vi "Basic Function Generator.vi"(3 "offset":dbl format="%0.2p", 4 "square wave duty cycle (%)":dbl=50.0 format="%0.2f", 5 "reset signal":bool, 6 "sampling info":cluster{"Fs":dbl, "#s":dbl}={"Fs"=1000.0, "#s"=1000.0} {"Fs" format="%.2p"}, 7 "signal type":T1(ring), 8 "error in (no error)":errorcluster, 9 "phase":dbl format="%.2p", 10 "amplitude":dbl=1.0 format="%0.2p", 11 "frequency":dbl=10.0 format="%0.2p") -> (0 "error out":errorcluster, 1 "phase out":dbl format="%.2p", 2 "signal out":waveform(dbl))   [LabVIEW 2020, in "NI_MABase.lvlib"]
doc: "Creates an output waveform based on <B>signal type</B>."
uses:
  NI_MABase.lvlib
  NI_AALBase.lvlib
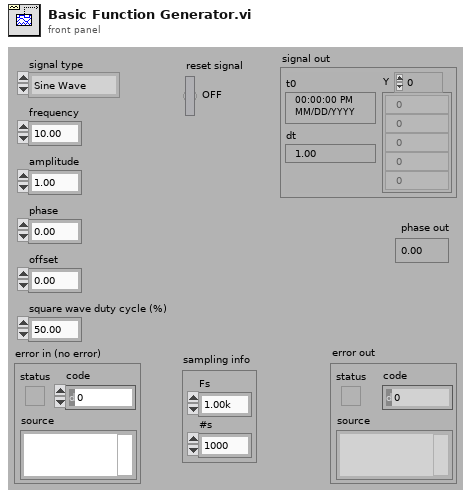
[diagram p1: front panel]
types:
  T1 = enum16{"Sine Wave", "Triangle Wave", "Square Wave", "Sawtooth Wave"}
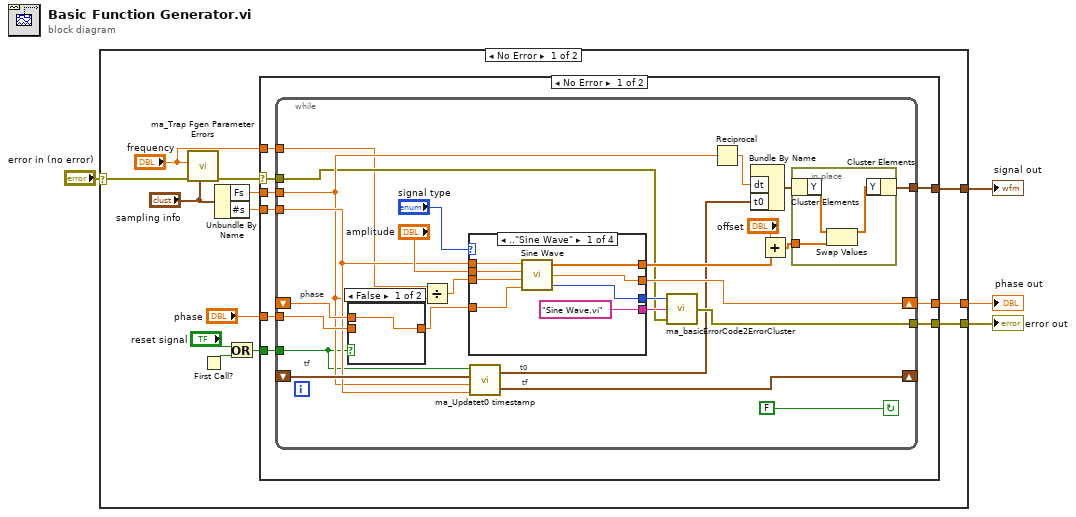
[diagram p0: block diagram]
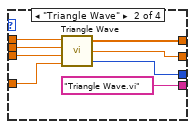
[diagram p2: hidden frame]
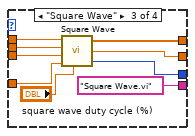
[diagram p3: hidden frame]
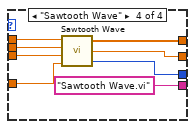
[diagram p4: hidden frame]
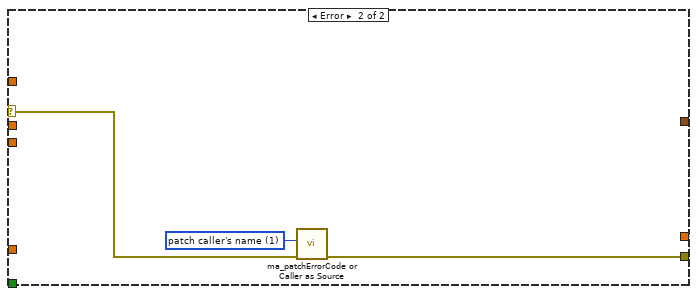
[diagram p6: hidden frame]
diagram:
  n1 = case shown="No Error" "error in (no error)" {
    selector: "error in (no error)" -> [w8 w94]
    tunnel: [w17 w94] -> w4
    tunnel: [w6 _] -> w2
    tunnel: [w5 _] -> w1
    frame No Error {
      n2 = call "ma_Trap Fgen Parameter Errors.vi"("Sampling info"="sampling info", "error in (no error)"=w8, "frequency"="frequency") -> ("error out"=w16:errorcluster)  [unwired: 8 in]
      n3 = First Call?() -> (First Call?: T/F=w11:bool)
      n4 = Unbundle By Name("sampling info") -> ("Fs"=w13:dbl, "#s"=w12:dbl)
      n5 = Or(x="reset signal", y=w11) -> (x .or. y?=w9:bool)
      n6 = case shown="No Error" w16 {
        selector: w16 -> [w20 w92]
        tunnel: [w26 w93] -> w5
        tunnel: [w25 w91] -> w17
        tunnel: "phase" -> [w24 _]
        tunnel: w13 -> [w23 _]
        tunnel: w12 -> [w22 _]
        tunnel: w9 -> [w21 _]
        tunnel: [w18 _] -> w6
        tunnel: "frequency" -> [w19 _]
        frame No Error {
          n7 = while {
            tunnel: w20 -> [w35]
            tunnel: w21 -> [w38]
            tunnel: w22 -> [w40]
            tunnel: w23 -> [w39]
            tunnel: w24 -> [w49]
            tunnel: [w34] -> w25
            shift-left: _ -> [w51]
            shift-right: [w41] -> w26
            shift-left: _ -> [w50]
            shift-right: [w29] -> _
            tunnel: w19 -> [w32]
            tunnel: [w27] -> w18
            stop <- FALSE continue-if-true
            # "tf"
            # "t0"
            # "phase"
            # "tf"
            n8 = case shown="False" w38 {
              tunnel: w51 -> [w88 _]
              tunnel: [w88 w89] -> w43
              tunnel: w49 -> [_ w89]
              frame False {
              }
              frame True {
              }
            }
            n9 = Divide(x=w32, y=w39) -> (x/y=w46:dbl)
            n10 = case shown="..\"Sine Wave\"" "signal type" {
              tunnel: w46 -> [w62 w70 w79 w87]
              tunnel: "amplitude" -> [w61 w69 w78 w86]
              tunnel: w40 -> [w60 w68 w77 w85]
              tunnel: w43 -> [w59 w67 w76 w84]
              tunnel: [w58 w66 w75 w83] -> w41
              tunnel: [w57 w65 w74 w82] -> w45
              tunnel: ["Sine Wave.vi" ("subVI Name") "Triangle Wave.vi" ("subVI Name") "Square Wave.vi" ("subVI Name") "Sawtooth Wave.vi" ("subVI Name")] -> w37
              tunnel: [w56 w64 w72 w80] -> w36
              frame .."Sine Wave" {
                n11 = call "Sine Wave.vi"("samples"=w60, "amplitude"=w61, "frequency"=w62, "phase in"=w59) -> ("sine wave"=w57:dbl[], "phase out"=w58:dbl, "error"=w56:i32)  [unwired: 1 in]
              }
              frame "Triangle Wave" {
                n12 = call "Triangle Wave.vi"("samples"=w68, "amplitude"=w69, "frequency"=w70, "phase in"=w67) -> ("triangle wave"=w65:dbl[], "phase out"=w66:dbl, "error"=w64:i32)  [unwired: 1 in]
              }
              frame "Square Wave" {
                n13 = call "Square Wave.vi"("samples"=w77, "amplitude"=w78, "frequency"=w79, "duty cycle (%)"="square wave duty cycle (%)", "phase in"=w76) -> ("square wave"=w74:dbl[], "phase out"=w75:dbl, "error"=w72:i32)  [unwired: 1 in]
              }
              frame "Sawtooth Wave" {
                n14 = call "Sawtooth Wave.vi"("samples"=w85, "amplitude"=w86, "frequency"=w87, "phase in"=w84) -> ("sawtooth wave"=w82:dbl[], "phase out"=w83:dbl, "error"=w80:i32)  [unwired: 1 in]
              }
            }
            n15 = call "ma_Updatet0 timestamp.vi"("samples"=w40, "sampling rate (S/s)"=w39, "tf previous"=w50, "Reset Generation"=w38) -> ("tf new"=w29:timestamp, "t0"=w33:timestamp)
            n16 = call "ma_basicErrorCode2ErrorCluster.vi"("error in (no error)"=w35, "subVI name"=w37, "Error Code"=w36) -> ("error out"=w34:errorcluster)
            n17 = Reciprocal(x=w39) -> (1/x=w47:dbl)
            n18 = Bundle By Name("dt"=w47, "t0"=w33) -> (w28:waveform(dbl))  [unwired: 1 in]
            n19 = Add(x="offset", y=w45) -> (x+y=w30:dbl[])
            n20 = in-place {
              in-place-border: w30 -> [w52]
              n21 = in-place-cluster #1(w28) -> ("Y"=w54:dbl[])
              n22 = Swap Values(12:w54, 14:w52) -> (1:w53:dbl[])  [unwired: 1 in, 1 out]
              n23 = in-place-cluster #1("Y"=w53) -> (w27:waveform(dbl))
            }
          }
        }
        frame Error {
          w90 = u16 1 items=["patch error code", "patch caller's name"] ("operation")
          w93 = 0.0  # phase out
          n24 = call "ma_patchErrorCode or Caller as Source.vi"("error in (no error)"=w92, "operation"=w90) -> ("error out"=w91:errorcluster)  [unwired: 9 in]
        }
      }
    }
    frame Error {
    }
  }
  "error out" <- w4
  "signal out" <- w2
  "phase out" <- w1
